vi "7L23-c-pi_Ccpc_init.vi"(2 "Pénalité (e)":T1, 3 "Pièce e":T2) -> (0 "Pénalité (s)":T1, 1 "Pièce s":T2)   [LabVIEW 2010, in "lv_07.lvlib"]
uses:
  lv_07.lvlib
  c_pi_wilson.ctl
  c_pi_penalite.ctl
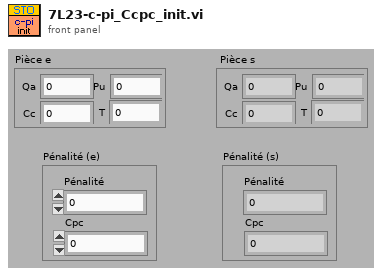
[diagram p1: front panel]
types:
  T1 = typedef "lv_07.lvlib/c_pi_penalite.ctl" = cluster{"Pénalité":dbl, "Cpc":dbl}
  T2 = typedef "lv_07.lvlib/c_pi_wilson.ctl" = cluster{"T":dbl, "Pu":dbl, "Qa":dbl, "Cc":dbl}
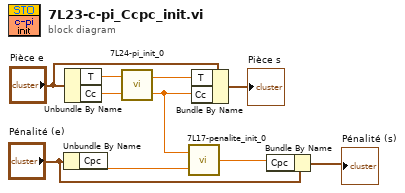
[diagram p0: block diagram]
diagram:
  n1 = Unbundle By Name("Pénalité (e)") -> ("Cpc"=w10:dbl)
  n2 = Unbundle By Name("Pièce e") -> ("T"=w9:dbl, "Cc"=w8:dbl)
  n3 = call "7L24-pi_init_0.vi"("Cc"=w8, "T"=w9) -> ("Cc init"=w5:dbl, "T init"=w6:dbl)
  n4 = call "7L17-penalite_init_0.vi"("Ccpc"=w10, "Cc"=w5) -> ("Ccpc init"=w3:dbl)
  n5 = Bundle By Name(cluster="Pièce e", "T"=w6, "Cc"=w5) -> (→"Pièce s":T2)
  n6 = Bundle By Name(cluster="Pénalité (e)", "Cpc"=w3) -> (→"Pénalité (s)":T1)
